vi "rtin_getNslMux.vi"(8 "error in":errorcluster, 10 "mux_mode":i32, 11 "connection ID":i32) -> (0 "error out":errorcluster, 3 "connection ID":i32)   [LabVIEW 2016]
doc: "get the axis the NSL multiplexer is set to"
panel:
  out "params_cluster":cluster{"mux_mode":i32}
  in  "Params_cluster":cluster{"integer":i32}
  in  "results_cluster":cluster{"errNo":i32}
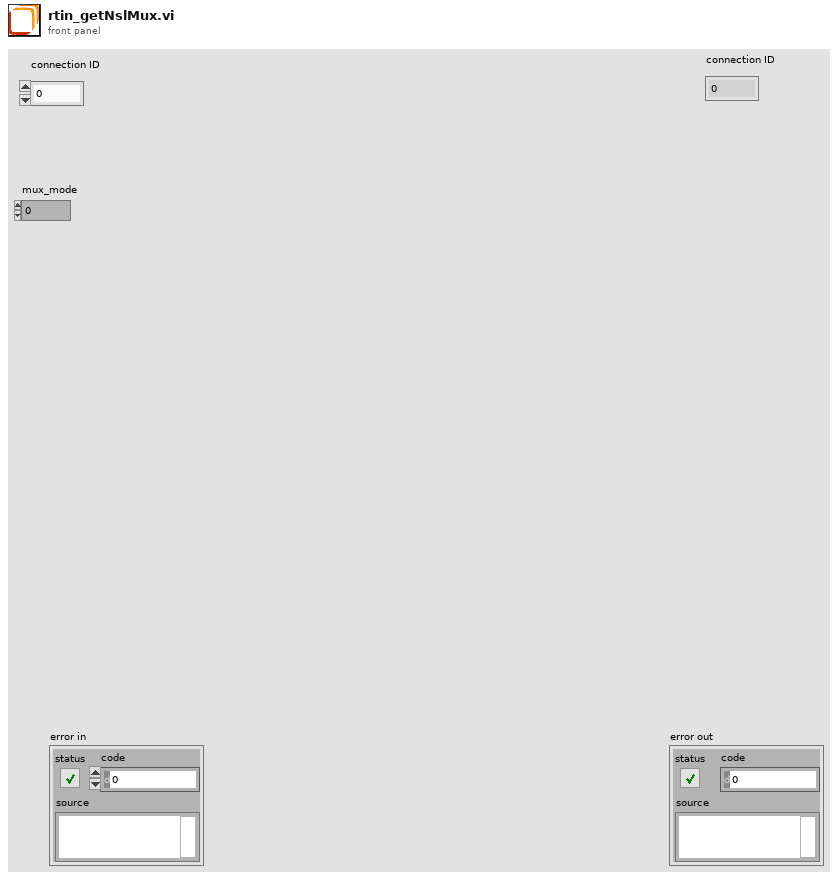
[diagram p1: front panel]
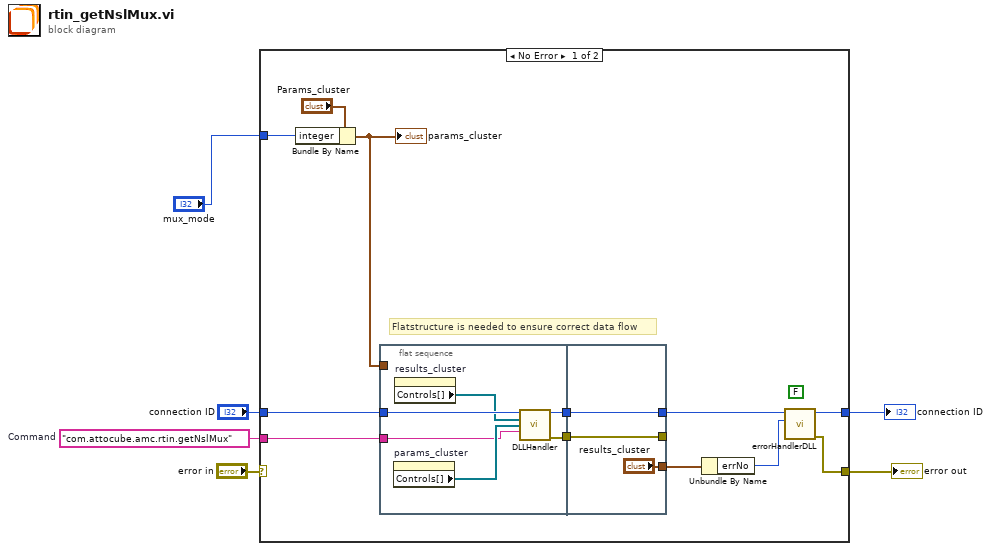
[diagram p0: block diagram]
diagram:
  w4 = "com.attocube.amc.rtin.getNslMux"  # Command
  n1 = case shown="No Error" "error in" {
    selector: "error in" -> [_ w29]
    tunnel: [w8 w29] -> w6
    tunnel: "connection ID" -> [w18 w28]
    tunnel: w4 -> [w15 _]
    tunnel: [w10 w28] -> w2
    tunnel: "mux_mode" -> [w7 _]
    frame No Error {
      (unwired) FALSE ("show popup")
      # "Flatstructure is needed to ensure correct data flow"
      n2 = Bundle By Name(cluster="Params_cluster", "integer"=w7) -> (w13:cluster{"integer":i32})
      "params_cluster" <- w13
      n3 = flat-sequence {
        tunnel: w18 -> [w24]
        tunnel: w15 -> [w21]
        tunnel: [w20] -> w14
        tunnel: w13 -> [_]
        tunnel: [w19] -> w11
        tunnel: ["results_cluster"] -> w17
        tunnel: [w27] -> w12
        tunnel: [w25] -> _
        tunnel: w14 -> [w25]
        tunnel: w11 -> [w27]
        frame #0 {
          n4 = property on="params_cluster" class="Clust (strict)"() -> ("Controls[]"=w22:refnum<vi>[])  [unwired: 2 in, 2 out]
          n5 = property on="results_cluster" class="Clust (strict)"() -> ("Controls[]"=w23:refnum<vi>[])  [unwired: 2 in, 2 out]
          n6 = call "DLLHandler.vi"("connection ID"=w24, "results_cluster"=w23, "params_cluster"=w22, "method"=w21) -> ("connection ID out"=w19:i32, "error"=w20:errorcluster)  [unwired: 10 in]
        }
        frame #1 {
        }
      }
      n7 = Unbundle By Name(w17) -> ("errNo"=w9:i32)
      n8 = call "errorHandlerDLL.vi"("error number"=w9, "connection ID"=w12) -> ("error out"=w8:errorcluster, "connection ID"=w10:i32)  [unwired: 8 in]
    }
    frame Error {
    }
  }
  "error out" <- w6
  "connection ID" <- w2
